vi "enqueue_DAQ.vi"(8 "error in":errorcluster, 9 "flush?":bool, 10 "elements in":T1[](array[typedef]), 11 "queue in":refnum<queue>) -> (0 "error out":errorcluster, 3 "queue out":refnum<queue>)   [LabVIEW 2015]
uses:
  Type Definitions/notifier_elements_DAQ.ctl
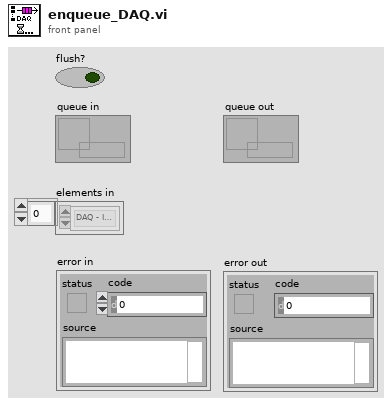
[diagram p1: front panel]
types:
  T1 = typedef "notifier_elements_DAQ.ctl" = enum16{"DAQ - Initialize", "DAQ - Pause", "DAQ - Run", "DAQ - Quit"}
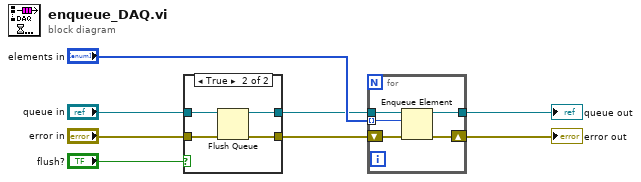
[diagram p0: block diagram]
diagram:
  n1 = case shown="True" "flush?" {
    tunnel: "queue in" -> [w10 w14]
    tunnel: [w10 w13] -> w3
    tunnel: "error in" -> [w9 w12]
    tunnel: [w9 w11] -> w1
    frame False {
    }
    frame True {
      n2 = Flush Queue(queue=w14, error in (no error)=w12) -> (queue out=w13:refnum<queue>, error out=w11:errorcluster)  [unwired: 1 out]
    }
  }
  n3 = for {
    tunnel: w3 -> [w18]
    shift-right: [w17] -> w8
    shift-left: w1 -> [w19]
    tunnel: "elements in" -> [w16] mode=indexing
    tunnel: [w15] -> w7
    n4 = Enqueue Element(queue=w18, element=w16, error in (no error)=w19) -> (queue out=w15:refnum<queue>, error out=w17:errorcluster)  [unwired: 1 in, 1 out]
  }
  "queue out" <- w7
  "error out" <- w8
